vi "dvp Vi Set Strobe Driver.vi"(10 "StrobeDriver":u32(ring) items=["FRAME_DURATION", "TIMER_LOGIC", "SENSOR_STROBE"], 11 "handle":u32) -> (3 "function return":u32(ring))   [LabVIEW 2018, in "LabViewDVPCamera.lvlib"]
doc: "LabviewDvp2Api dvpStatus dvpViSetStrobeDriver(dvpHandle handle, dvpStrobeDriver StrobeDriver);"
uses:
  LabViewDVPCamera.lvlib
  LabViewDVPCamera/LabViewDVPCamera.dll
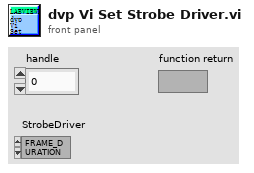
[diagram p1: front panel]
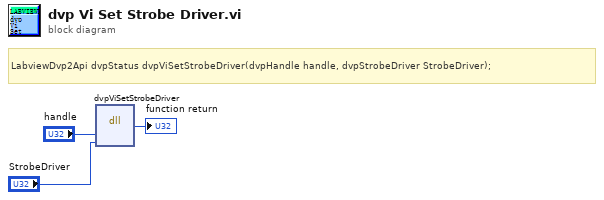
[diagram p0: block diagram]
diagram:
  # "LabviewDvp2Api dvpStatus dvpViSetStrobeDriver(dvpHandle handle, dvpStrobeDriver StrobeDriver);"
  n1 = dll-call lib="C:/Program Files (x86)/DVP2 Labview cn 64/Sample/LabViewDVPCamera/LabViewDVPCamera.*" fn="dvpViSetStrobeDriver"("handle"="handle", "StrobeDriver"="StrobeDriver") -> (→"function return":u32)  [unwired: 5 in, 2 out]
